vi "Add graph.vi"(8 "error in (no error)":errorcluster, 10 "Combo Box":string(combo)="Kinetics", 11 "Control-Client in":refnum<class "Control-Client.lvclass">) -> (0 "error out":errorcluster, 3 "Control-Client out":refnum<class "Control-Client.lvclass">)   [LabVIEW 2019, in "Control-Client.lvclass"]
uses:
  Control-Client.lvclass
  Control-Client.lvclass/Control-Client.ctl
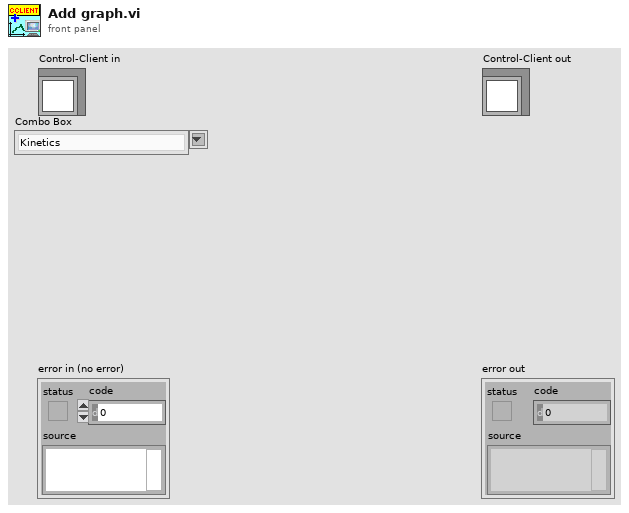
[diagram p1: front panel]
types:
  T1 = cluster{"waves slider":refnum<vi>, "times slider":refnum<vi>}
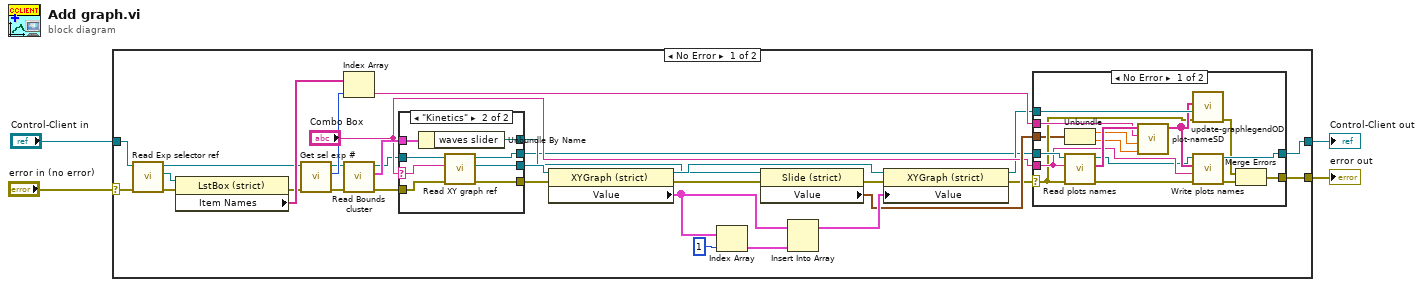
[diagram p0: block diagram]
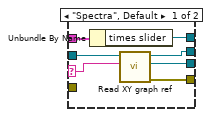
[diagram p2: hidden frame]
diagram:
  n1 = case shown="No Error" "error in (no error)" {
    selector: "error in (no error)" -> [w5 w70]
    tunnel: [w29 w70] -> w3
    tunnel: [w28 w69] -> w1
    tunnel: "Control-Client in" -> [w22 w69]
    frame No Error {
      n2 = call "Read Exp selector ref.vi"("error in (no error)"=w5, "Control-Client in"=w22) -> ("error out"=w23:errorcluster, "Exp selector ref"=w27:refnum<vi>, "Control-Client out"=w7:refnum<class "Control-Client.lvclass">)  [unwired: 7 in]
      n3 = property class="LstBox (strict)"(reference=w27, error in=w23) -> (error out=w8:errorcluster, "Item Names"=w26:string[])  [unwired: 1 out]
      n4 = call "Get sel exp #.vi"("error in (no error)"=w8, "Control-Client in"=w7) -> ("error out"=w9:errorcluster, "Exp sel #"=w25:i32, "Control-Client out"=w10:refnum<class "Control-Client.lvclass">)  [unwired: 7 in]
      n5 = Index Array(array=w26, index=w25) -> (element=w24:string)
      n6 = call "Read Bounds cluster.vi"("error in (no error)"=w9, "Control-Client in"=w10) -> ("error out"=w13:errorcluster, "Bounds cluster"=w21:T1, "Control-Client out"=w16:refnum<class "Control-Client.lvclass">)  [unwired: 7 in]
      n7 = case shown="\"Kinetics\"" "Combo Box" {
        selector: "Combo Box" -> [w42 w45]
        tunnel: [w40 w50] -> w18
        tunnel: [w39 w49] -> w30
        tunnel: w16 -> [w41 w48]
        tunnel: w21 -> [w38 w47]
        tunnel: [w37 w46] -> w17
        tunnel: [w36 w44] -> w14
        tunnel: w13 -> [_ w43]
        frame "Spectra", Default {
          n8 = Unbundle By Name(w38) -> ("times slider"=w37:refnum<vi>)
          n9 = call "Read XY graph ref.vi"("Combo Box"=w42, "Control-Client in"=w41) -> ("error out"=w39:errorcluster, "XY graph ref"=w40:refnum<vi>, "Control-Client out"=w36:refnum<class "Control-Client.lvclass">)  [unwired: 7 in]
        }
        frame "Kinetics" {
          n10 = Unbundle By Name(w47) -> ("waves slider"=w46:refnum<vi>)
          n11 = call "Read XY graph ref.vi"("error in (no error)"=w43, "Combo Box"=w45, "Control-Client in"=w48) -> ("error out"=w49:errorcluster, "XY graph ref"=w50:refnum<vi>, "Control-Client out"=w44:refnum<class "Control-Client.lvclass">)  [unwired: 6 in]
        }
      }
      n12 = property class="XYGraph (strict)"(reference=w18, error in=w30) -> (reference out=w35:refnum<vi>, error out=w12:errorcluster, "Value"=w31:cluster{"Y":dbl[], "Y":dbl[]}[])
      n13 = Index Array(array=w31, index=1) -> (element=w33:cluster{"Y":dbl[], "Y":dbl[]})
      n14 = property class="Slide (strict)"(reference=w17, error in=w12) -> (error out=w11:errorcluster, "Value"=w20:cluster{dbl, dbl})  [unwired: 1 out]
      n15 = Insert Into Array(array=w31, new element=w33) -> (w32:cluster{"Y":dbl[], "Y":dbl[]}[])  [unwired: 1 in]
      n16 = property class="XYGraph (strict)"(reference=w35, error in=w11, "Value"=w32) -> (reference out=w15:refnum<vi>, error out=w6:errorcluster)
      n17 = case shown="No Error" w6 {
        selector: w6 -> [w57 w68]
        tunnel: [w55 w68] -> w29
        tunnel: w14 -> [w65 w67]
        tunnel: [w66 w67] -> w28
        tunnel: w24 -> [w62 _]
        tunnel: w20 -> [w54 _]
        tunnel: "Combo Box" -> [w61 _]
        tunnel: w15 -> [w60 _]
        frame No Error {
          n18 = Unbundle(w54) -> (w53:dbl, w52:dbl)
          n19 = call "Read plots names.vi"("error in (no error)"=w57, "Combo Box"=w61, "Control-Client in"=w65) -> ("error out"=w64:errorcluster, "Plots names"=w63:string[], "Control-Client out"=w51:refnum<class "Control-Client.lvclass">)  [unwired: 6 in]
          n20 = call "plot-nameSD.vi"("To"=w52, "from"=w53, "Item name"=w62, "plot names in"=w63) -> ("plot names out"=w59:string[])  [unwired: 7 in]
          n21 = call "update-graphlegendOD.vi"("error in (no error)"=w57, "XYGraph in"=w60, "plot names"=w59) -> ("error out"=w56:errorcluster)  [unwired: 7 in]
          n22 = call "Write plots names.vi"("error in (no error)"=w64, "Combo Box"=w61, "Plot names"=w59, "Control-Client in"=w51) -> ("error out"=w58:errorcluster, "Control-Client out"=w66:refnum<class "Control-Client.lvclass">)  [unwired: 6 in]
          n23 = Merge Errors(w56, w58) -> (w55:errorcluster)
        }
        frame Error {
        }
      }
    }
    frame Error {
    }
  }
  "error out" <- w3
  "Control-Client out" <- w1
